vi "Restart LabVIEW.vi"() -> ()   [LabVIEW 2012, in "Application.lvlib"]
uses:
  Application.lvlib
panel:
  out "错误输出":errorcluster
  in  "错误输入（无错误）":errorcluster
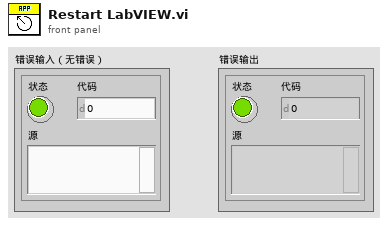
[diagram p1: front panel]
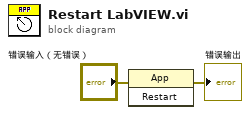
[diagram p0: block diagram]
diagram:
  n1 = invoke class="App" method="Restart"(error in="错误输入（无错误）") -> (error out=→"错误输出":errorcluster)  [unwired: 2 in, 2 out]
